vi "[SubVI]Torque_Conversion.vi"(6 "Left Alpha Angle":dbl, 7 "Right Alpha Angle":dbl, 8 "Left Torque In":dbl format="%#_13g", 9 "Right Torque In":dbl format="%#_13g") -> (0 "Left PWM":dbl, 1 "Right PWM":dbl, 2 "Left DIR":bool, 3 "Right DIR":bool, 4 "L.Current":dbl, 5 "R.Current":dbl)   [LabVIEW 2019]
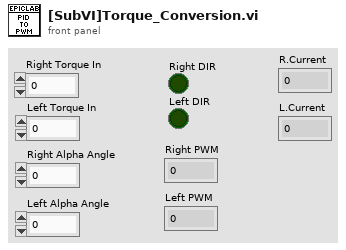
[diagram p1: front panel]
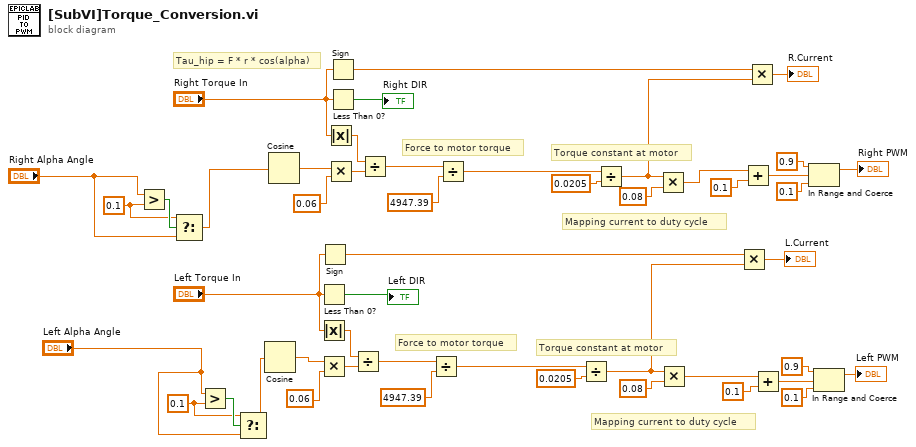
[diagram p0: block diagram]
diagram:
  w3 = 0.1 ("y")
  w7 = 0.1 ("y")
  # "Force to motor torque"
  # "Torque constant at motor"
  # "Mapping current to duty cycle"
  # "Tau_hip = F * r * cos(alpha)"
  # "Force to motor torque"
  # "Torque constant at motor"
  # "Mapping current to duty cycle"
  n1 = Greater?(x="Right Alpha Angle", y=w3) -> (0:w4:bool)
  n2 = Select(t=w3, s=w4, f="Right Alpha Angle") -> (s? t:f=w1:dbl)
  n3 = Greater?(x="Left Alpha Angle", y=w7) -> (0:w8:bool)
  n4 = Select(t=w7, s=w8, f="Left Alpha Angle") -> (s? t:f=w5:dbl)
  n5 = Cosine(x=w5) -> (cos(x)=w9:dbl)
  n6 = Cosine(x=w1) -> (cos(x)=w10:dbl)
  n7 = Less Than 0?(x="Left Torque In") -> (x < 0?=→"Left DIR":bool)
  n8 = Absolute Value(x="Left Torque In") -> (abs(x)=w44:dbl)
  n9 = Multiply(x=w9, y=0.06) -> (x*y=w37:dbl)
  n10 = Sign(1:"Left Torque In") -> (0:w16:dbl)
  n11 = Absolute Value(x="Right Torque In") -> (abs(x)=w39:dbl)
  n12 = Multiply(x=w10, y=0.06) -> (x*y=w36:dbl)
  n13 = Sign(1:"Right Torque In") -> (0:w18:dbl)
  n14 = Less Than 0?(x="Right Torque In") -> (x < 0?=→"Right DIR":bool)
  n15 = Divide(x=w44, y=w37) -> (x/y=w45:dbl)
  n16 = Divide(x=w39, y=w36) -> (x/y=w33:dbl)
  n17 = Divide(x=w45, y=4947.39) -> (x/y=w46:dbl)
  n18 = Divide(x=w33, y=4947.39) -> (x/y=w41:dbl)
  n19 = Divide(x=w46, y=0.0205) -> (x/y=w12:dbl)
  n20 = Divide(x=w41, y=0.0205) -> (x/y=w13:dbl)
  n21 = Multiply(x=w13, y=0.08) -> (x*y=w19:dbl)
  n22 = Multiply(x=w12, y=0.08) -> (x*y=w11:dbl)
  n23 = Multiply(x=w16, y=w12) -> (x*y=→"L.Current":dbl)
  n24 = Add(x=w19, y=0.1) -> (x+y=w29:dbl)
  n25 = Multiply(x=w18, y=w13) -> (x*y=→"R.Current":dbl)
  n26 = Add(x=w11, y=0.1) -> (x+y=w30:dbl)
  n27 = In Range and Coerce(upper limit=0.9, x=w29, lower limit=0.1) -> (coerced(x)=→"Right PWM":dbl)  [unwired: 1 out]
  n28 = In Range and Coerce(upper limit=0.9, x=w30, lower limit=0.1) -> (coerced(x)=→"Left PWM":dbl)  [unwired: 1 out]
